vi "wirteFile.vi"(6 "base path":path, 7 "dataIn":string, 11 "name":path) -> ()   [LabVIEW 2021]
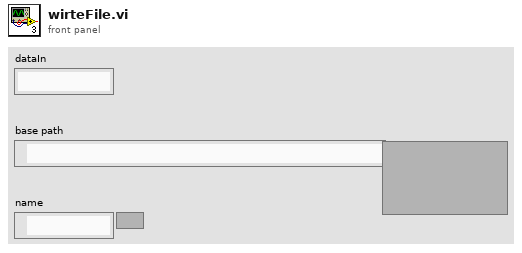
[diagram p1: front panel]
types:
  T1 = enum16{"open", "replace", "create", "open or create", "replace or create", "replace or create with confirmation"}
  T2 = enum16{"big-endian, network order", "native, host order", "little-endian"}
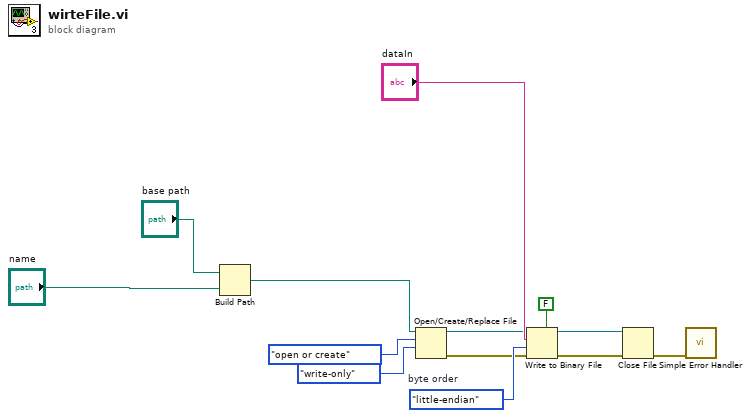
[diagram p0: block diagram]
diagram:
  w12 = T2."little-endian"  # byte order
  n1 = Build Path(base path="base path", name or relative path="name") -> (appended path=w3:path)
  n2 = Open/Create/Replace File(file path (use dialog)=w3, operation (0:open)=T1."open or create", access (0:read/write)=enum16{"read/write", "read-only", "write-only"}."write-only") -> (refnum out=w2:refnum<file>, error out=w9:errorcluster)  [unwired: 3 in, 1 out]
  n3 = Write to Binary File(file (use dialog)=w2, data="dataIn", error in=w9, 5:FALSE ("prepend array or string size? (T)"), 9:w12) -> (refnum out=w6:refnum<file>, error out=w7:errorcluster)  [unwired: 1 in, 1 out]
  n4 = Close File(refnum=w6, error in=w7) -> (error out=w8:errorcluster)  [unwired: 1 out]
  n5 = call <vilib>:"Simple Error Handler.vi"("error in (no error)"=w8) -> ()  [unwired: 4 in, 5 out]
